vi "test Get and Set Cache.vi"(8 "error in (no error)":errorcluster, 11 "TestCase in":refnum<class "Framework Tests.lvclass">) -> (0 "error out":errorcluster, 3 "TestCase out":refnum<class "Framework Tests.lvclass">)   [LabVIEW 2017, in "Framework Tests.lvclass"]
uses:
  Framework Tests.lvclass
  Engine/Classes/Transfer Group/Transfer Group.lvclass
  Engine/Classes/Transfer/Transfer.lvclass
  Mock Framework Class/Mock Framework.lvclass
  C:/github/data-sharing-framework/Data Sharing Framework Core/Engine/Classes/Framework/Framework.lvclass
  Engine/Classes/Framework/Framework.lvclass/Framework.ctl
  Engine/Classes/Cache/Cache.lvclass/Cache.ctl
  <vilib>/addons/_JKI Toolkits/VI Tester/TestCase.llb/TestCase.lvclass
  Engine/Classes/Cache/Cache.lvclass
  Engine/Classes/Framework/Framework.lvclass
  C:/Program Files (x86)/National Instruments/LabVIEW 2017/vi.lib/addons/_JKI Toolkits/VI Tester/TestCase.llb/TestCase.lvclass
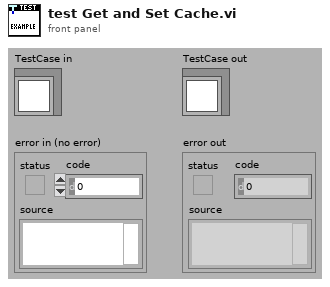
[diagram p1: front panel]
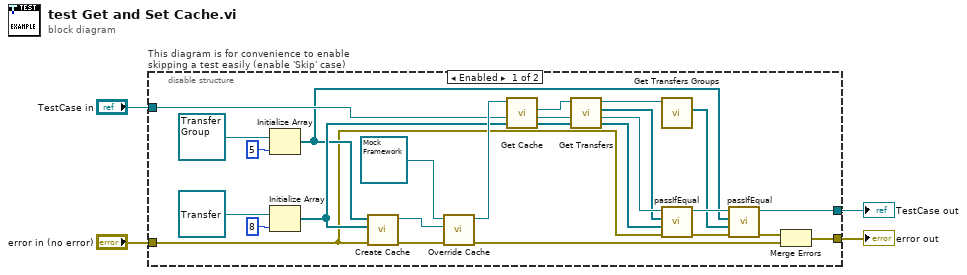
[diagram p0: block diagram]
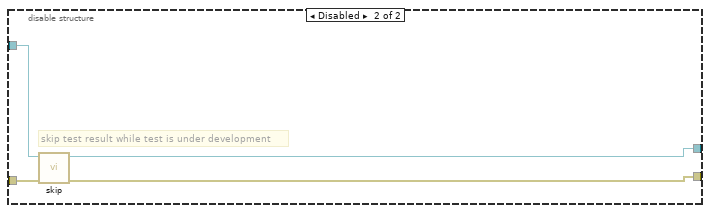
[diagram p2: hidden frame]
diagram:
  n1 = disable-structure "This diagram is for convenience to enable skipping a test easily (enable 'Skip' case)" shown="Enabled" {
    disable-tunnel: "TestCase in" -> [w18 w30]
    disable-tunnel: [w13 w28] -> w1
    disable-tunnel: [w9 w29] -> w3
    disable-tunnel: "error in (no error)" -> [w7 w27]
    frame Enabled {
      n2 = Initialize Array(refnum<class "Transfer Group.lvclass"> refnum ("DSF Core.lvlib:Transfer Group"), 5 ("dimension size")) -> (w12:refnum<class "Transfer Group.lvclass">[])
      n3 = Initialize Array(refnum<class "Transfer.lvclass"> refnum ("DSF Core.lvlib:Transfer"), 8 ("dimension size")) -> (w16:refnum<class "Transfer.lvclass">[])
      n4 = call "Create Cache.vi"("error in (no error)"=w7, "Transfers"=w16, "Transfers Groups"=w12) -> ("error out"=w10:errorcluster, "Cache out"=w21:refnum<class "Cache.lvclass">)  [unwired: 7 in]
      n5 = call "Override Cache.vi"("error in (no error)"=w10, "Cache"=w21, "Mock Framework in"=refnum<class "Mock Framework.lvclass"> refnum) -> ("error out"=w8:errorcluster, "Mock Framework out"=w20:refnum<class "Mock Framework.lvclass">)  [unwired: 7 in]
      n6 = call "Get Cache.vi"("Framework in"=w20) -> ("Cache"=w6:refnum<class "Cache.lvclass">)  [unwired: 9 in, 1 out]
      n7 = call "Get Transfers.vi"("Cache in"=w6) -> ("Transfers"=w17:refnum<class "Transfer.lvclass">[], "Cache out"=w5:refnum<class "Cache.lvclass">)  [unwired: 9 in]
      n8 = call "Get Transfers Groups.vi"("Cache in"=w5) -> ("Transfers Groups"=w11:refnum<class "Transfer Group.lvclass">[])  [unwired: 9 in, 1 out]
      n9 = call-dynamic "passIfEqual.vi"("error in (no error)"=w7, "y"=w16, "x"=w17, "TestCase in"=w18) -> ("error out"=w19:errorcluster, "TestCase out"=w14:refnum<class "Framework Tests.lvclass">)  [unwired: 6 in]
      n10 = call-dynamic "passIfEqual.vi"("error in (no error)"=w19, "y"=w11, "x"=w12, "TestCase in"=w14) -> ("error out"=w15:errorcluster, "TestCase out"=w13:refnum<class "Framework Tests.lvclass">)  [unwired: 6 in]
      n11 = Merge Errors(w15, w8) -> (w9:errorcluster)
    }
    frame Disabled {
      # "skip test result while test is under development"
      n12 = call <vilib>:"skip.vi"("error in (no error)"=w27, "TestCase in"=w30) -> ("error out"=w29:errorcluster, "TestCase out"=w28:refnum<class "Framework Tests.lvclass">)  [unwired: 8 in]
    }
  }
  "error out" <- w3
  "TestCase out" <- w1
